vi "RT Sync Monitor.vi"(8 "error in (no error)":errorcluster) -> (2 "x/y":dbl)   [LabVIEW 2022 SP3]
uses:
  RT Controls/RT All Loop Status.ctl
  <instrlib>/niSync/niSync.llb/niSync Initialize (Default).vi
  RT Global.vi
panel:
  out "Error Out":errorcluster
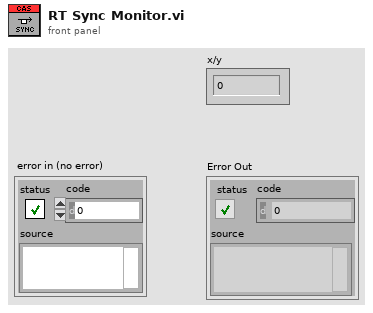
[diagram p1: front panel]
types:
  T1 = typedef "RT All Loop Status.ctl" = enum16{"AI", "AO", "DI", "DO", "TC", "Strain", "ACC", "RT", "Log", "Seq", "Sync"}
  T2 = enum16{"Init", "Read 'All'", "Read 'n'", "Read '1'", "Write '1'", "Write 'n'", "Write 'All'"}
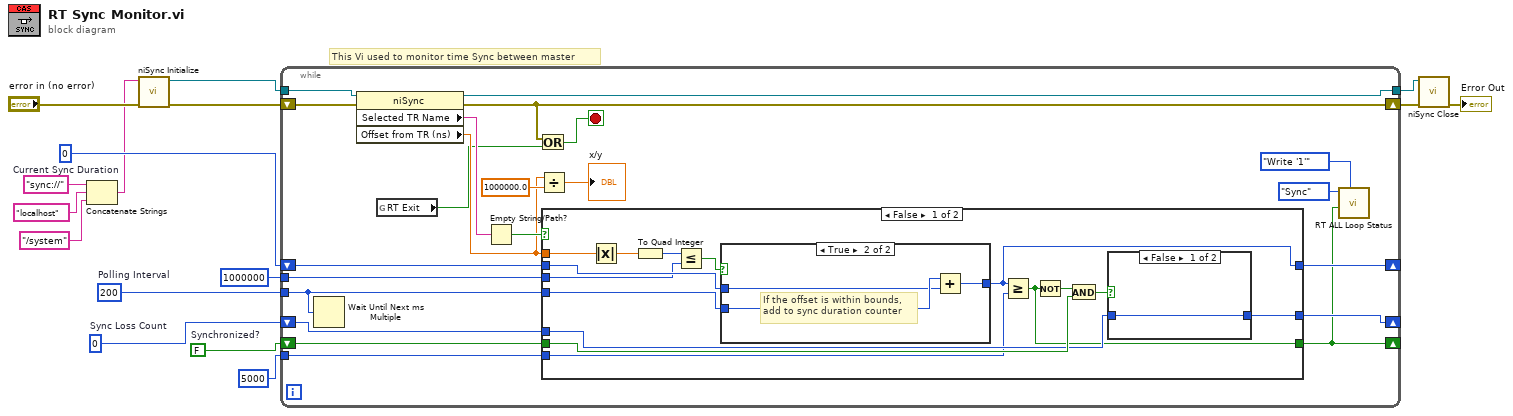
[diagram p0: block diagram]
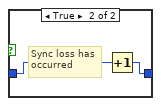
[diagram p2: hidden frame]
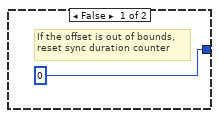
[diagram p3: hidden frame]
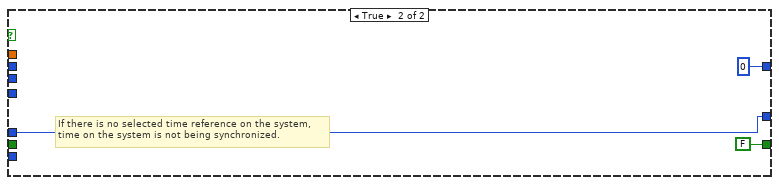
[diagram p4: hidden frame]
diagram:
  w8 = u32 200  # Polling Interval
  w9 = u32 0  # Sync Loss Count
  w10 = FALSE  # Synchronized?
  w15 = u32 0  # Current Sync Duration
  # "This Vi used to monitor time Sync between master"
  n1 = Concatenate Strings("sync://" ("string"), "localhost" ("string"), "/system" ("string")) -> (w2:string)
  n2 = call-poly <instrlib>:"niSync Initialize.vi"("error in (no error)"="error in (no error)", "resource name"=w2) -> ("error out"=w14:errorcluster, "instrument handle out"=w16:refnum<k15>)  [unwired: 8 in]
  n3 = while {
    tunnel: w16 -> [w25]
    tunnel: [w38] -> w12
    shift-right: [w29] -> _
    shift-left: w15 -> [w33]
    tunnel: i64 1000000 ("Max Offset") -> [w34]
    shift-right: [w27] -> w11
    shift-left: w14 -> [w37]
    shift-right: [w17] -> _
    shift-left: w10 -> [w36]
    shift-right: [w28] -> _
    shift-left: w9 -> [w35]
    tunnel: w8 -> [w21]
    tunnel: u32 5000 ("Min Sync Duration") -> [w32]
    stop <- w26 stop-if-true
    n4 = Wait Until Next ms Multiple(millisecond multiple=w21) -> ()  [unwired: 1 out]
    n5 = property class="niSync"(reference=w25, error in=w37) -> (reference out=w38:refnum<k15>, error out=w27:errorcluster, "Selected TR Name"=w30:string, "Offset from TR (ns)"=w23:dbl)
    n6 = global read "RT Global.vi" "RT Exit"() -> (w20:bool)
    n7 = Empty String/Path?(string/path=w30) -> (empty?=w31:bool)
    n8 = Or(x=w27, y=w20) -> (x .or. y?=w26:bool)
    n9 = Divide(x=w23, y=1000000.0 ("x")) -> (x/y=→"x/y":dbl)
    n10 = case shown="False" w31 {
      tunnel: w36 -> [w52 _]
      tunnel: w35 -> [w49 w62]
      tunnel: w23 -> [w48 _]
      tunnel: w34 -> [w41 _]
      tunnel: [w43 u32 0] -> w29
      tunnel: [w42 FALSE] -> w17
      tunnel: w33 -> [w47 _]
      tunnel: w21 -> [w46 _]
      tunnel: [w45 w62] -> w28
      tunnel: w32 -> [w44 _]
      frame False {
        n11 = Absolute Value(x=w48) -> (abs(x)=w39:dbl)
        n12 = To Quad Integer(1:w39) -> (0:w40:i64)
        n13 = Less Or Equal?(x=w40, y=w41) -> (x <= y?=w53:bool)
        n14 = case shown="True" w53 {
          tunnel: [u32 0 w60] -> w43
          tunnel: w46 -> [_ w59]
          tunnel: w47 -> [_ w58]
          frame False {
            # "If the offset is out of bounds,\nreset sync duration counter"
          }
          frame True {
            # "If the offset is within bounds,\nadd to sync duration counter"
            n15 = Add(x=w59, y=w58) -> (x+y=w60:u32)
          }
        }
        n16 = Greater Or Equal?(x=w43, y=w44) -> (x >= y?=w42:bool)
        n17 = Not(x=w42) -> (.not. x?=w51:bool)
        n18 = And(x=w51, y=w52) -> (x .and. y?=w50:bool)
        n19 = case shown="False" w50 {
          tunnel: w49 -> [w54 w56]
          tunnel: [w54 w55] -> w45
          frame False {
          }
          frame True {
            # "Sync loss has\noccurred"
            n20 = Increment(x=w56) -> (x+1=w55:u32)
          }
        }
      }
      frame True {
        # "If there is no selected time reference on the system,\ntime on the system is not being synchronized."
      }
    }
    n21 = call "RT ALL Loop Status.vi"("Option"=T2."Write '1'", "Status"=w17, "Loop"=RT_All_Loop_Status."Sync") -> ()  [unwired: 6 in, 3 out]
  }
  n22 = call <instrlib>:"niSync Close.vi"("error in (no error)"=w11, "instrument handle"=w12) -> ("error out"=→"Error Out":errorcluster)  [unwired: 9 in]
